vi "Fieldscan - plot data.vi"(6 "Data acquisition interval (s)":dbl format="%#.1f", 8 "error in (no error)":errorcluster, 10 "Data":T2, 11 "Action":T1) -> (0 "error out":errorcluster)   [LabVIEW 2019]
doc: "Nicolas Weiss - EPFL - IPHYS 2019\n----"
uses:
  Controls/Data to save cluster.ctl
  Controls/Plot data action.ctl
panel:
  out "Graph 2":cluster{"Field":dbl[], "Y-axis data":dbl[]}(graph)
  out "Graph 1":cluster{"Field":dbl[], "Y data":dbl[]}(graph)
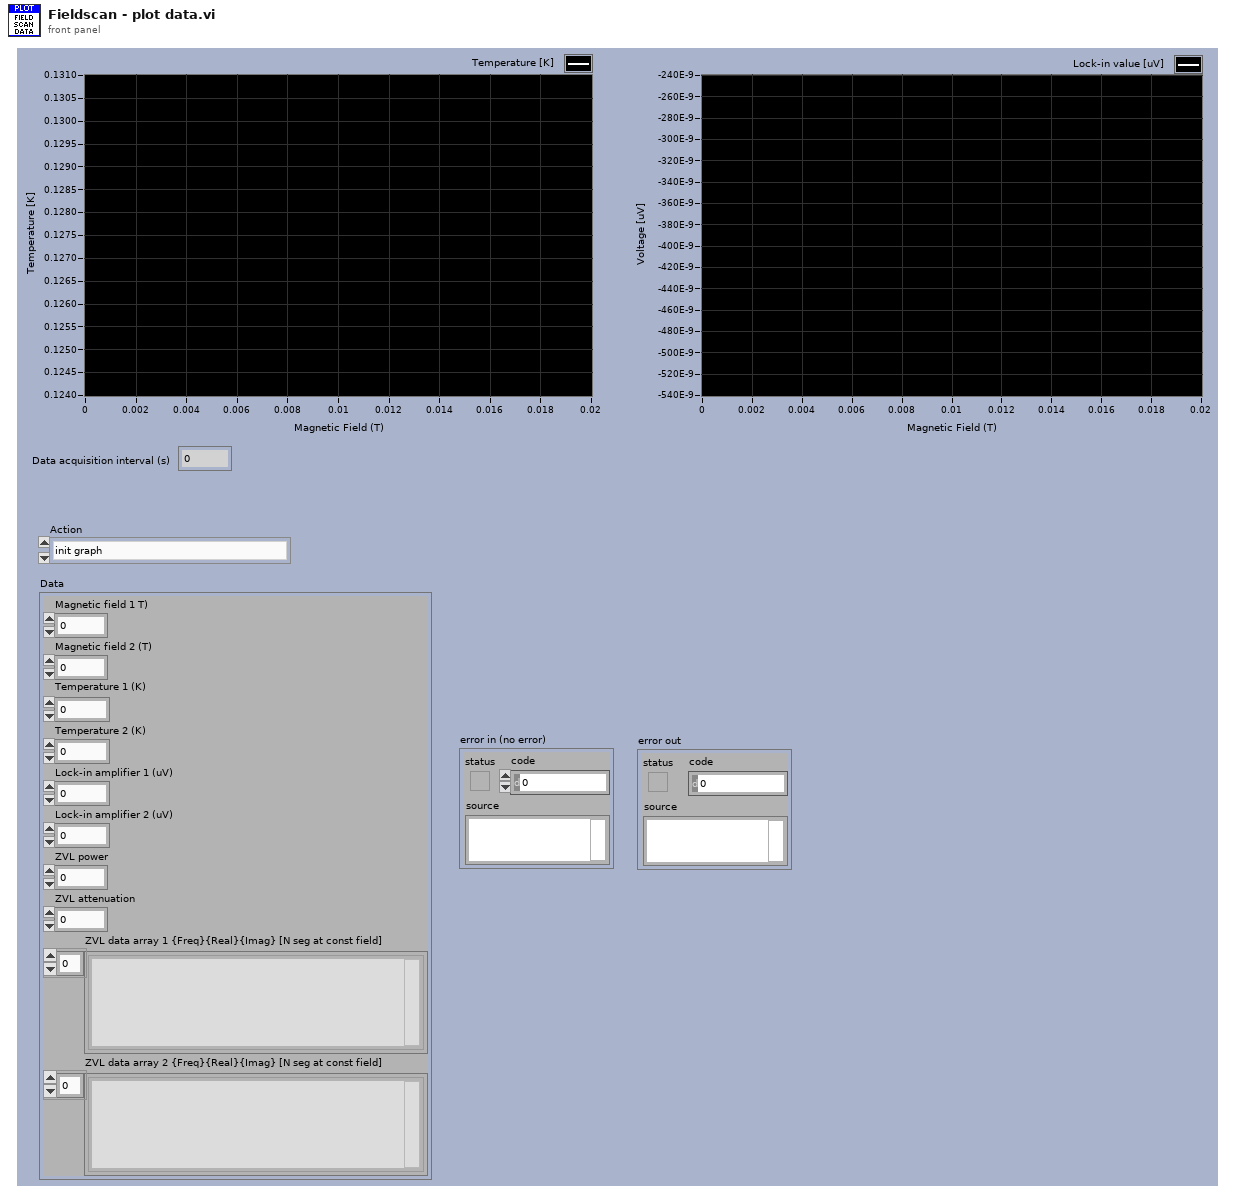
[diagram p1: front panel]
types:
  T1 = typedef "Plot data action.ctl" = enum16{"init graph", "Append data"}
  T2 = typedef "Data to save cluster.ctl" = cluster{"Magnetic field 1 T)":dbl, "Magnetic field 2 (T)":dbl, "Temperature 1 (K)":dbl, "Temperature 2 (K)":dbl, "Lock-in amplifier 1 (uV)":dbl, "Lock-in amplifier 2 (uV)":dbl, "ZVL power":dbl, "ZVL attenuation":dbl, "ZVL data array 1 {Freq}{Real}{Imag} [N seg at const field]":string[], "ZVL data array 2 {Freq}{Real}{Imag} [N seg at const field]":string[]}
  T3 = enum32{"Invalid", "Standard", "Closed", "Hidden", "Minimized", "Maximized"}
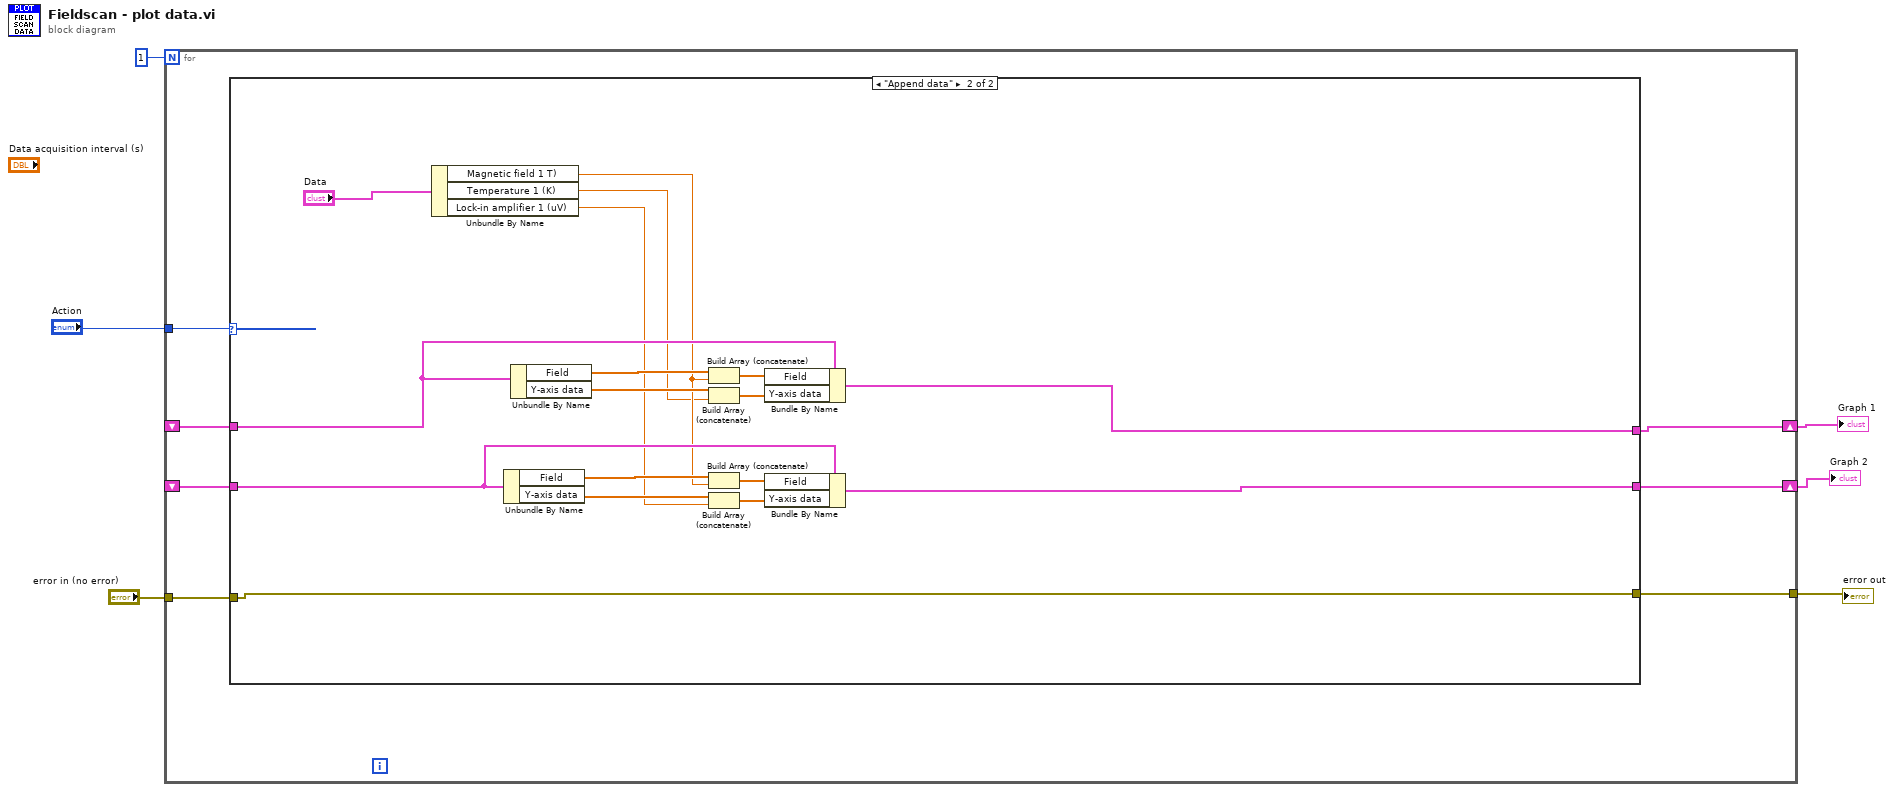
[diagram p0: block diagram]
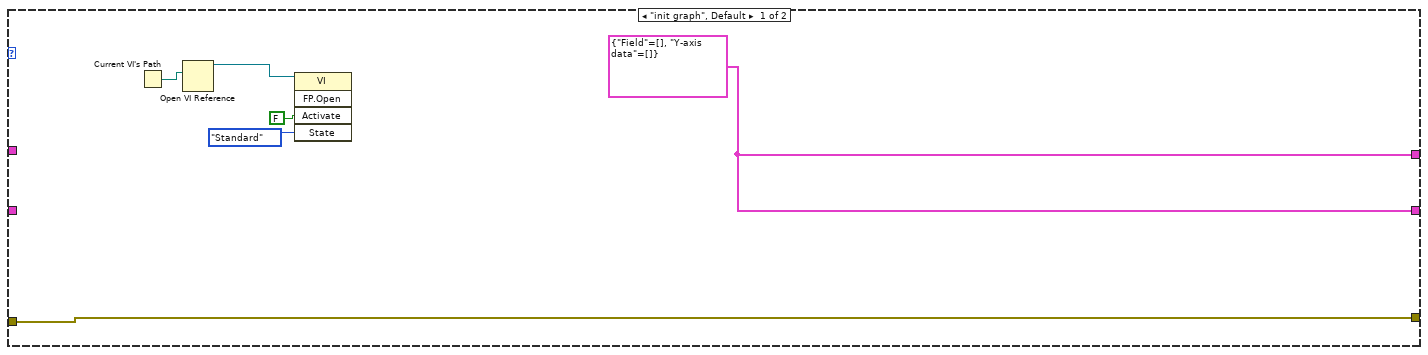
[diagram p2: hidden frame]
diagram:
  n1 = for {
    N: 1 -> [_]
    tunnel: "Action" -> [w13]
    tunnel: "error in (no error)" -> [w12]
    tunnel: [w11] -> w4
    shift-right: [w9] -> w2
    shift-left: _ -> [w10]
    shift-right: [w7] -> w1
    shift-left: _ -> [w8]
    n2 = case shown="\"Append data\"" w13 {
      tunnel: w12 -> [w19 w24]
      tunnel: [w19 w24] -> w11
      tunnel: w10 -> [_ w27]
      tunnel: [w18 w26] -> w9
      tunnel: w8 -> [_ w23]
      tunnel: [w18 w25] -> w7
      frame "init graph", Default {
        w18 = cluster{"Field":dbl[], "Y-axis data":dbl[]} {"Field"=[], "Y-axis data"=[]}
        n3 = Current VI's Path() -> (path=w16:path)
        n4 = Open VI Reference(vi path=w16) -> (vi reference=w17:refnum<vi>)  [unwired: 5 in, 1 out]
        n5 = invoke class="VI" method="FP.Open"(reference=w17, "Activate"=FALSE ("Activate?"), "State"=T3."Standard") -> ()  [unwired: 2 in, 5 out]
      }
      frame "Append data" {
        n6 = Unbundle By Name("Data") -> ("Magnetic field 1 T)"=w22:dbl, "Temperature 1 (K)"=w21:dbl, "Lock-in amplifier 1 (uV)"=w20:dbl)
        n7 = Unbundle By Name(w23) -> ("Field"=w31:dbl[], "Y-axis data"=w30:dbl[])
        n8 = Unbundle By Name(w27) -> ("Field"=w35:dbl[], "Y-axis data"=w34:dbl[])
        n9 = Build Array (concatenate)(w35, w22) -> (w33:dbl[])
        n10 = Build Array (concatenate)(w34, w21) -> (w32:dbl[])
        n11 = Build Array (concatenate)(w31, w22) -> (w29:dbl[])
        n12 = Build Array (concatenate)(w30, w20) -> (w28:dbl[])
        n13 = Bundle By Name(cluster=w27, "Field"=w33, "Y-axis data"=w32) -> (w26:cluster{"Field":dbl[], "Y-axis data":dbl[]})
        n14 = Bundle By Name(cluster=w23, "Field"=w29, "Y-axis data"=w28) -> (w25:cluster{"Field":dbl[], "Y-axis data":dbl[]})
      }
    }
  }
  "error out" <- w4
  "Graph 1" <- w2
  "Graph 2" <- w1
